vi "Delete_SN.vi"(8 "error in (no error)":errorcluster caption="entrée d'erreur (pas d'erreur)", 11 "Class Creation_SN (Default) en entrée":refnum<class "Creation_SN Database (Default).lvclass">) -> (0 "error out":errorcluster caption="sortie d'erreur", 3 "Class Creation_SN (Default) en sortie":refnum<class "Creation_SN Database (Default).lvclass">)   [LabVIEW 2020, in "Library Instrument & Equipement.lvlib" / "Library Creation_SN.lvlib" / "Creation_SN Database (Default).lvclass"]
uses:
  Creation_SN Database (Default).lvclass
  Instrument/Instrument Firebase Altyor/Class Instrument Firebase Altyor.lvclass
  Creation_SN Database (Default).lvclass/Creation_SN Database (Default).ctl
  Firebase/Source/Firebase Recovery_SN/Firebase Recovery_SN.lvclass
  C:/Users/ngarcin/OneDrive - Altyor/Standard TB/Class/Firebase/Source/Firebase Driver/Firebase Driver.lvclass
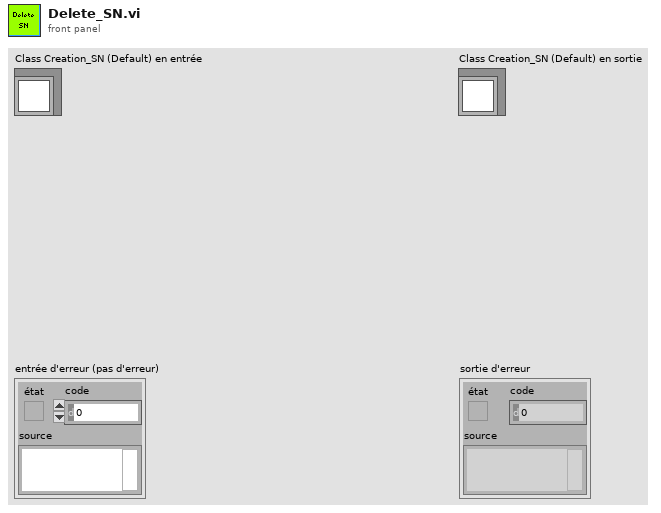
[diagram p1: front panel]
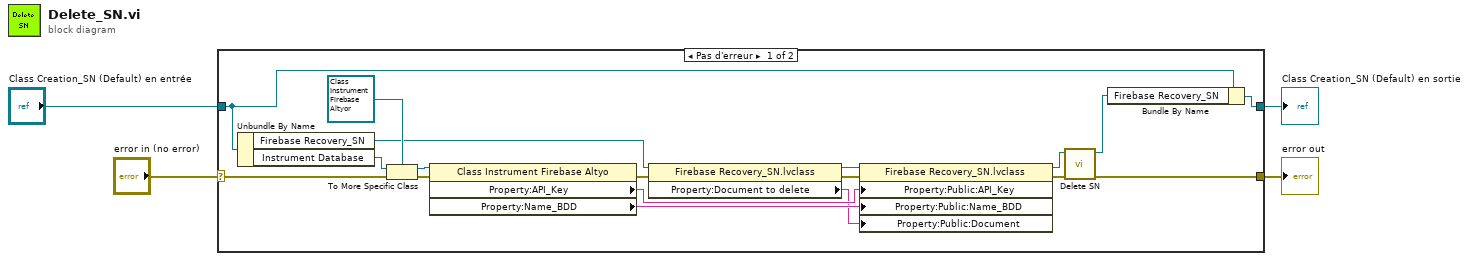
[diagram p0: block diagram]
diagram:
  n1 = case shown="Pas d'erreur" "error in (no error)" {
    selector: "error in (no error)" -> [w15 w24]
    tunnel: [w12 w24] -> w3
    tunnel: [w14 w23] -> w1
    tunnel: "Class Creation_SN (Default) en entrée" -> [w22 w23]
    frame No Error {
      n2 = Unbundle By Name(w22) -> ("Firebase Recovery_SN"=w9:refnum<class "Firebase Recovery_SN.lvclass">, "Instrument Database"=w16:refnum<class "Class Instrument (Default).lvclass">)
      n3 = To More Specific Class(target class=refnum<class "Class Instrument Firebase Altyor.lvclass"> refnum ("Library Instruments.lvlib:Class Instrument Firebase Altyor.lvclass"), reference=w16, error in=w15) -> (specific class reference=w19:refnum<class "Class Instrument Firebase Altyor.lvclass">, error out=w20:errorcluster)
      n4 = property class="Class Instrument Firebase Altyo"(reference=w19, error in=w20) -> (error out=w7:errorcluster, "Property:API_Key"=w18:string, "Property:Name_BDD"=w17:string)  [unwired: 1 out]
      n5 = property class="Firebase Recovery_SN.lvclass"(reference=w9, error in=w7) -> (reference out=w5:refnum<class "Firebase Recovery_SN.lvclass">, error out=w6:errorcluster, "Property:Document to delete"=w8:string)
      n6 = property class="Firebase Recovery_SN.lvclass"(reference=w5, error in=w6, "Property:Public:API_Key"=w18, "Property:Public:Name_BDD"=w17, "Property:Public:Document"=w8) -> (reference out=w10:refnum<class "Firebase Recovery_SN.lvclass">, error out=w13:errorcluster)
      n7 = call-dynamic "Delete SN.vi"("error in (no error)"=w13, "Firebase Benches en entrée"=w10) -> ("error out"=w12:errorcluster, "Firebase Benches en sortie"=w11:refnum<class "Firebase Recovery_SN.lvclass">)  [unwired: 8 in]
      n8 = Bundle By Name(cluster=w22, "Firebase Recovery_SN"=w11) -> (w14:refnum<class "Creation_SN Database (Default).lvclass">)
    }
    frame Error {
    }
  }
  "error out" <- w3
  "Class Creation_SN (Default) en sortie" <- w1
